vi "ChangeManipulator.vi"(6 "error in":errorcluster, 8 "Manipulator":u16(ring) items=["DriveA"=1, "DriveB"=2], 9 "VISA resource In":refnum<visa-resource-name>) -> (0 "error out":errorcluster, 3 "VISA resource name out":refnum<visa-resource-name>)   [LabVIEW 2016]
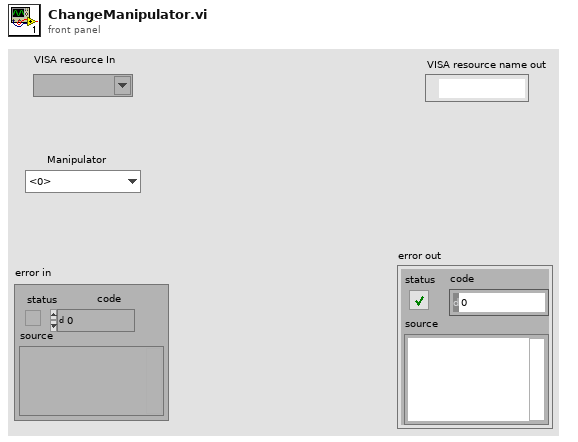
[diagram p1: front panel]
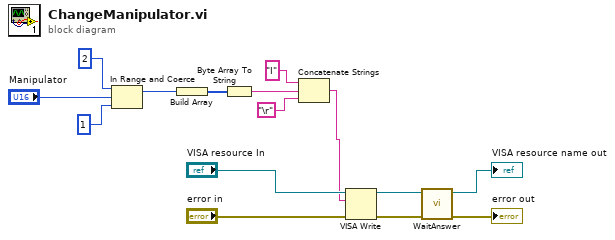
[diagram p0: block diagram]
diagram:
  n1 = In Range and Coerce(upper limit=u16 2, x="Manipulator", lower limit=u16 1) -> (coerced(x)=w3:u16)  [unwired: 1 out]
  n2 = Build Array(w3) -> (w6:u16[])
  n3 = Byte Array To String(unsigned byte array=w6) -> (string=w5:string)
  n4 = Concatenate Strings("I" ("string"), w5, "\r") -> (w7:string)
  n5 = VISA Write(VISA resource name="VISA resource In", write buffer=w7, error in (no error)="error in") -> (VISA resource name out=w13:refnum<visa-resource-name>, error out=w11:errorcluster)  [unwired: 1 out]
  n6 = call "WaitAnswer.vi"("error in (no error)"=w11, "VISA resource name in"=w13) -> ("error out"=→"error out":errorcluster, "VISA resource name out"=→"VISA resource name out":refnum<visa-resource-name>)  [unwired: 4 in]
